vi "Test Copy from Pixmap Offset.vi"(8 "error in (no error)":errorcluster, 11 "Test Case In":refnum<class "01_Image.lvclass">) -> (0 "error out":errorcluster, 3 "Test Case Out":refnum<class "01_Image.lvclass">)   [LabVIEW 2020, in "test.lvlib" / "01_Image.lvclass"]
uses:
  01_Image.lvclass
  C:/Program Files (x86)/National Instruments/LabVIEW 2026/vi.lib/Astemes/LUnit/Test Case.lvclass
  image/ARGB Colour.ctl
  <vilib>/Astemes/LUnit/Test Case.lvclass/Test Case.ctl
  image/New Image (ARGB Preallocated).vi
  image/Copy Pixmap to Image (ARGB Flatten Mask).vi
  4993e8ee-a06a-463a-9684-69129f64d5ce.vi
  image/New Image (ARGB Preallocated).vi/3321fa97-f432-4e1e-8db9-a0df79aed21b.vi
  image/ARGB Colour to U32 Pixel Value.vi
  image/Copy Pixmap to Image (ARGB Flatten Mask).vi/7d03ccf7-b889-4e8d-9f2a-57831e73dbde.vi
  <vilib>/Astemes/LUnit/Core/LUnit Test Case/Private/Append Pass Result.vi
  <vilib>/Astemes/LUnit/Core/LUnit Test Case/Private/Append Fail Result.vi
  4993e8ee-a06a-463a-9684-69129f64d5ce.vi/9c5d11cd-9439-4240-a1ee-d9baace9c924.vi
  image/FixPixmap.vi
  <vilib>/Astemes/LUnit/Core/LUnit Test Case/Private/Run In UI.vi
  image/Default8bitColourMap.vi
  <vilib>/Utility/error.llb/Clear Errors.vi
  <vilib>/Utility/error.llb/Error Cluster From Error Code.vi
  image/image.lvlib
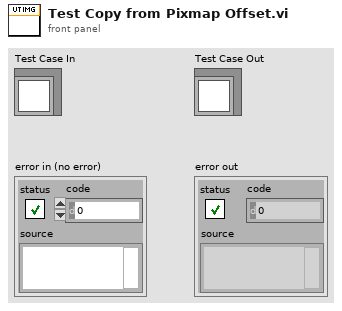
[diagram p1: front panel]
types:
  T1 = cluster{"Width":i16, "Style":enum32{"Solid", "Dash", "Dot", "DashDot", "DashDotDot"}}
  T2 = typedef "image.lvlib/ARGB Colour.ctl" = cluster{"Alpha":u8, "RGB":u32}
  T3 = cluster{"left":i16, "top":i16, "right":i16, "bottom":i16}
  T4 = typedef "imagedata.ctl" = cluster{"image type":i32, "image depth":i32, "image":u8[], "mask":u8[], "colors":u32[], "Rectangle":cluster{"left":i16, "top":i16, "right":i16, "bottom":i16}}
  T5 = typedef "image.lvlib/ARGB Image.ctl" = refnum<data-value>
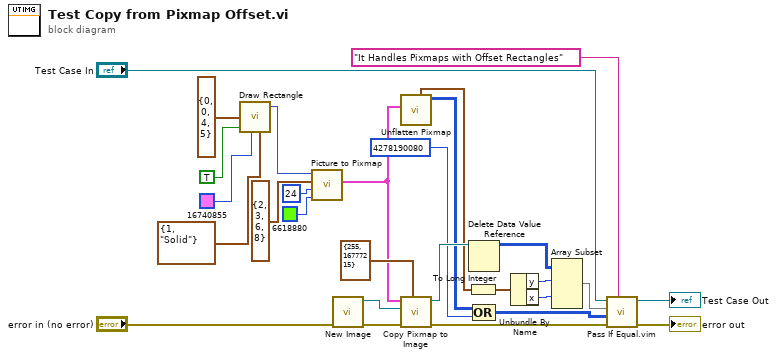
[diagram p0: block diagram]
diagram:
  n1 = call <vilib>:"Draw Rectangle.vi"("rect"=T3 {"left"=0, "top"=0, "right"=4, "bottom"=5}, "fill?(F)"=TRUE, "color(black)"=u32 16740855, "pen"=T1 {"Width"=1, "Style"=enum."Solid"}) -> ("new picture"=w23:picture)  [unwired: 5 in]
  n2 = call <vilib>:"Picture to Pixmap.vi"("Background Color"=u32 6618880, "depth"=24, "rect"=T3 {"left"=2, "top"=3, "right"=6, "bottom"=8}, "picture"=w23) -> ("image data"=w14:T4)  [unwired: 6 in, 1 out]
  n3 = call-poly "New Image.vi"("error in (no error)"="error in (no error)") -> ("error out"=w2:errorcluster, "ARGB Image"=w18:T5)  [unwired: 9 in]
  n4 = call <vilib>:"Unflatten Pixmap.vi"("image data"=w14) -> ("24-bit pixmap"=w7:u32[][], "top left"=w11:cluster{"x":i16, "y":i16})  [unwired: 4 in, 5 out]
  n5 = call-poly "Copy Pixmap to Image.vi"("Colour (Default: Black)"=T2 {"Alpha"=255, "RGB"=16777215}, "error in (no error)"=w2, "ARGB Image Destination in"=w18, "Pixmap Image Data"=w14) -> ("error out"=w1:errorcluster, "ARGB Image Destination"=w13:T5)  [unwired: 6 in]
  n6 = To Long Integer(number=w11) -> (32bit integer=w8:cluster{"x":i32, "y":i32})
  n7 = Delete Data Value Reference(data value reference=w13) -> (data value=w12:u32[][])  [unwired: 1 in, 1 out]
  n8 = Compound Arithmetic op=OR(w7, u32 4278190080) -> (w5:u32[][])
  n9 = Unbundle By Name(w8) -> ("y"=w10:i32, "x"=w9:i32)
  n10 = Array Subset(array=w12, index (row)=w10, index (col)=w9) -> (w4:u32[][])  [unwired: 2 in]
  n11 = call "Pass If Equal.vim"("Description"="It Handles Pixmaps with Offset Rectangles", "error in (no error)"=w1, "Actual"=w5, "Expected"=w4, "LUnit Test Case In"="Test Case In") -> ("error out"=→"error out":errorcluster, "LUnit Test Case Out"=→"Test Case Out":refnum<class "01_Image.lvclass">)  [unwired: 5 in]
